vi "Set_4060_Watchdog_Timer.vi"(3 "Watchdog Timer  Seconds":i32 min=0 max=6553, 4 "Port Name":string="MainNetwork", 5 "Module Address":i32) -> (0 "Comment out":string, 1 "Reply":string, 2 "String to Write":string)   [LabVIEW 2018]
panel:
  # "Happy reply starts \"!\"\nUnhappy reply starts \"?\""
  # "\"0\" means Watchdog disabled"
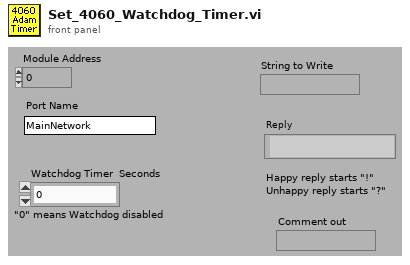
[diagram p1: front panel]
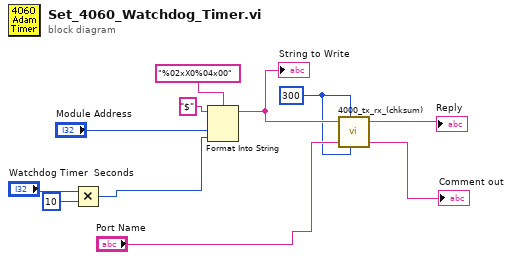
[diagram p0: block diagram]
diagram:
  w1 = u32 300 ("Timeout/ms")
  n1 = Multiply(x="Watchdog Timer  Seconds", y=10) -> (x*y=w6:i32)
  n2 = Format Into String(format string="%02xX0%04x00", initial string="$", "Module Address", w6) -> (resulting string=w5:string)  [unwired: 1 in, 1 out]
  "String to Write" <- w5
  n3 = call "4000_tx_rx_(chksum).vi"("Write String"=w5, "Timeout/ms"=w1, "Port Name"="Port Name", "Timeout/ms Short"=w1) -> ("Read"=→"Reply":string, "Comment out"=→"Comment out":string)  [unwired: 1 in, 1 out]
